vi "WASH simulated console.vi"(8 "error in (no error)":errorcluster) -> (0 "error out":errorcluster)   [LabVIEW 2015]
doc: "simulated console mimics ilustration from specification.\n\n[Covers: UI1]"
uses:
  type defs/WASH UI to CTRL commands.ctl
  type defs/WASH UI to CTRL message.ctl
  type defs/WASH CTRL to UI commands.ctl
  type defs/Wash CTRL to UI message.ctl
  type defs/WASH indicators.ctl
  type defs/WASH error levels.ctl
  type defs/WASH step selection buttons.ctl
panel:
  out "Abort":bool
  in  "Vehicle position simulation":i32(slide) scale=0.0..4.0
  out "time remaining":dbl format="%0#6.2f"
  out "vehicle out of position":bool
  out "wash indicators":T1
  out "Wash entry":bool
  in  "Start":bool
  in  "Wash step selection":T2
  # "[Covers: UI2]"
  # "[Covers: UI3]"
  # "[Covers: UI3A]\n[Covers: UI3A1]\n[Covers: UI3A2]\n[Covers: UI3A3]"
  # "[Covers: UI3B]\n[Covers: UI3B1]"
  # "[Covers: UI2A]"
  # "[Covers: UI2B]"
  # "[Covers: UI3C]\n[Covers: UI3C1]\n[Covers: UI3C2]"
  # "[Covers: UI3D]\n[Covers: UI3D1]"
  # "[Covers: UI4]"
  # "Entry"
  # "Station 1"
  # "Station 2"
  # "Station 3"
  # "Exit"
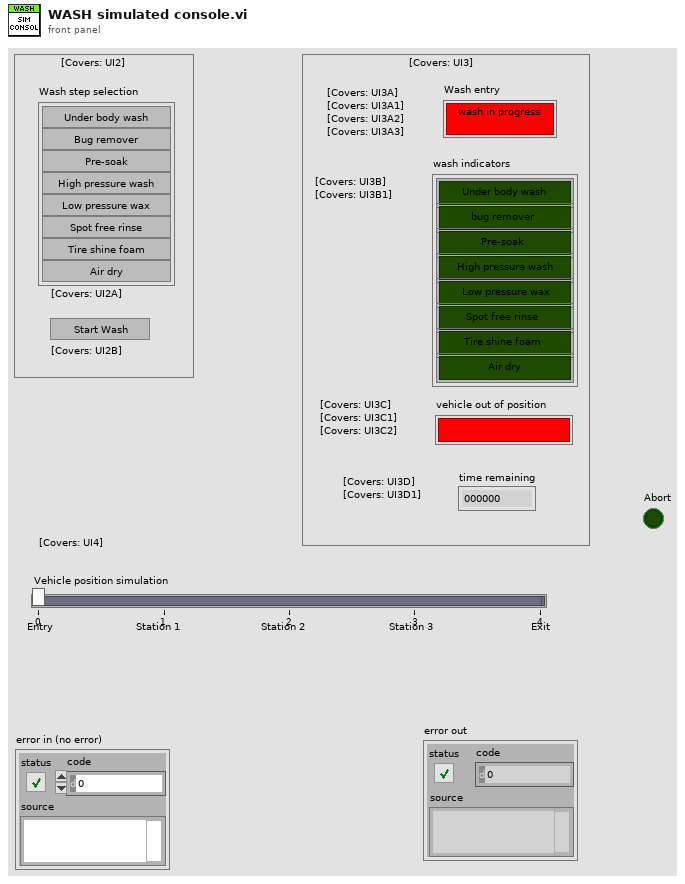
[diagram p1: front panel]
types:
  T1 = typedef "WASH indicators.ctl" = cluster{"Under body wash":bool, "bug remover":bool, "Pre-soak":bool, "High pressure wash":bool, "Low pressure wax":bool, "Spot free rinse":bool, "Tire shine foam":bool, "Air dry":bool}
  T2 = typedef "WASH step selection buttons.ctl" = cluster{"Under body wash":bool, "Bug remover":bool, "Pre-soak":bool, "High pressure wash":bool, "Low pressure wax":bool, "Spot free rinse":bool, "Tire shine foam":bool, "Air dry":bool}
  T3 = typedef "WASH UI to CTRL message.ctl" = cluster{"command":T4, "data":variant}
  T4 = typedef "WASH UI to CTRL commands.ctl" = enum16{"start button pushed", "vehicle position changed"}
  T5 = typedef "Wash CTRL to UI message.ctl" = cluster{"command":T6, "data":variant}
  T6 = typedef "WASH CTRL to UI commands.ctl" = enum16{"enable controls", "set start button value", "update vehicle out of pos", "update wash indicators", "update timing", "set vehicle position entry", "abort"}
  T7 = typedef "WASH error levels.ctl" = enum16{"minor", "wash cycle", "system"}
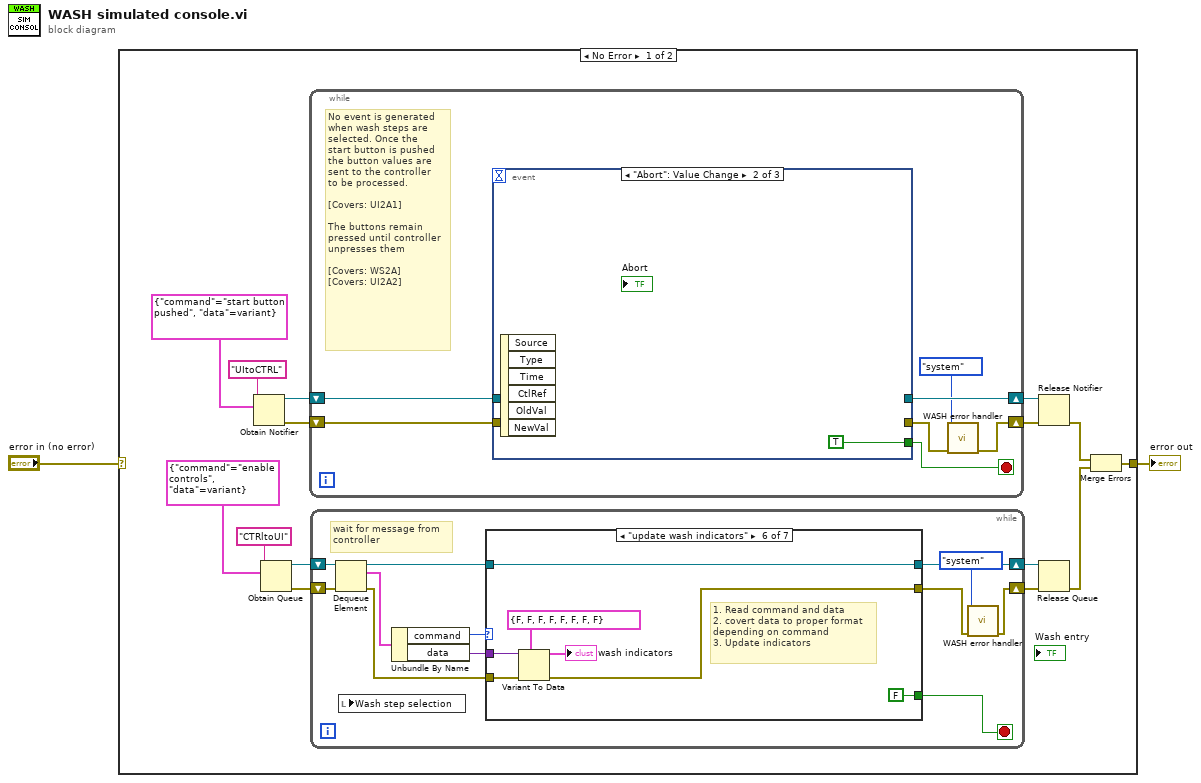
[diagram p0: block diagram]
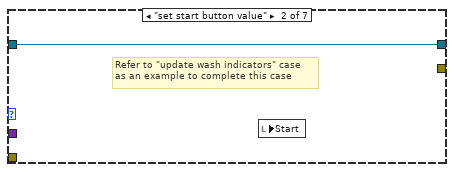
[diagram p3: hidden frame]
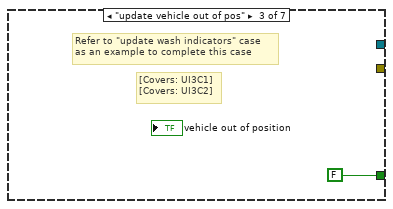
[diagram p4: hidden frame]
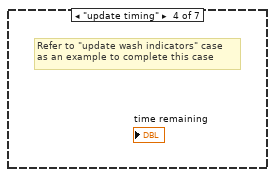
[diagram p5: hidden frame]
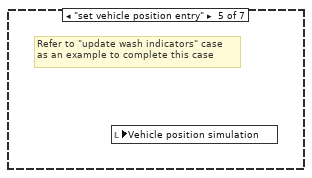
[diagram p6: hidden frame]
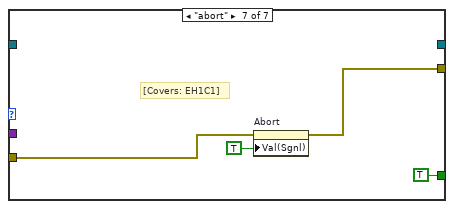
[diagram p7: hidden frame]
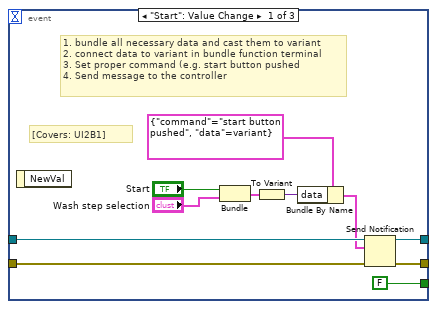
[diagram p8: hidden frame]
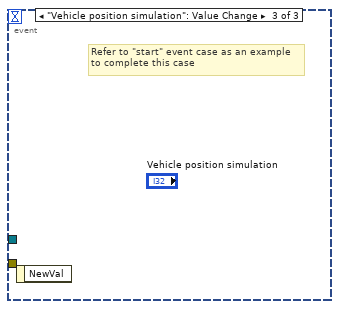
[diagram p9: hidden frame]
diagram:
  n1 = case shown="No Error" "error in (no error)" {
    selector: "error in (no error)" -> [_ w62]
    tunnel: [w3 w62] -> w1
    frame No Error {
      n2 = Obtain Notifier(name (unnamed)="UItoCTRL", notification data type=T3 {"command"=enum."start button pushed", "data"=variant} ("UI to CTRL message")) -> (notifier out=w17:refnum<notifier>, error out=w16:errorcluster)  [unwired: 2 in, 1 out]
      n3 = Obtain Queue(name (unnamed)="CTRltoUI", element data type=T5 {"command"=enum."enable controls", "data"=variant} ("CTRL to UI message")) -> (queue out=w12:refnum<queue>, error out=w11:errorcluster)  [unwired: 3 in, 1 out]
      n4 = while {
        shift-right: [w46] -> w15
        shift-left: w16 -> [w48]
        shift-right: [w47] -> w14
        shift-left: w17 -> [w49]
        stop <- w43 stop-if-true
        # "No event is generated\nwhen wash steps are\nselected. Once the\nstart button is pushed\nthe button values are\nsent to the controller\nto be processed.\n\n[Covers: UI2A1]\n\nThe buttons remain\npressed until controller\nunpresses them\n\n[Covers: WS2A]\n[Covers: UI2A2]"
        n5 = event shown="[1] \"Abort\": Value Change" {
          selector: _ -> [_ _ _]
          dyn-events: _ -> [_ _ _]
          timeout: _ -> [_ _ _]
          tunnel: w49 -> [w60 _ _]
          tunnel: [w59 _ _] -> w45
          tunnel: w48 -> [w58 _ _]
          tunnel: [w57 _ _] -> w47
          tunnel: [FALSE TRUE _] -> w43
          event "Start": Value Change {
            # "[Covers: UI2B1]"
            # "1. bundle all necessary data and cast them to variant\n2. connect data to variant in bundle function terminal\n3. Set proper command (e.g. start button pushed\n4. Send message to the controller"
            n6 = event-data() -> ()  [unwired: 1 in, 1 out]
            n7 = Bundle("Start"="Start", "Wash step selection"="Wash step selection") -> (w53:cluster{"Start":bool, "Wash step selection":T2})  [unwired: 1 in]
            n8 = To Variant(anything=w53) -> (Variant=w52:variant)
            n9 = Bundle By Name(cluster=T3 {"command"=enum."start button pushed", "data"=variant} ("notification"), "data"=w52) -> (w51:T3)
            n10 = Send Notification(notification=w51, notifier=w60, error in (no error)=w58) -> (notifier out=w57:refnum<notifier>, error out=w59:errorcluster)
          }
          event "Abort": Value Change {
            n11 = event-data() -> ()  [unwired: 1 in, 6 out]
          }
          event "Vehicle position simulation": Value Change {
            # "Refer to \"start\" event case as an example\nto complete this case"
            n12 = event-data() -> ()  [unwired: 1 in, 1 out]
          }
        }
        n13 = call "WASH error handler.vi"("error in (no error)"=w45, "error levels"=WASH_error_levels."system") -> ("error out"=w46:errorcluster)  [unwired: 7 in, 2 out]
      }
      n14 = while {
        shift-right: [w27] -> w7
        shift-left: w12 -> [w29]
        shift-right: [w20] -> w6
        shift-left: w11 -> [w28]
        stop <- w21 stop-if-true
        # "wait for message from\ncontroller"
        n15 = Dequeue Element(queue=w29, error in (no error)=w28) -> (queue out=w26:refnum<queue>, element=w25:T5, error out=w22:errorcluster)  [unwired: 1 in, 1 out]
        n16 = local read "Wash step selection"() -> ()  [unwired: 1 in]
        n17 = Unbundle By Name(w25) -> ("command"=w24:T6, "data"=w23:variant)
        n18 = case shown="\"update wash indicators\"" w24 {
          tunnel: [_ w30 _ _ _ w33 _] -> w27
          tunnel: w26 -> [_ w30 _ _ _ w33 _]
          tunnel: w23 -> [_ _ _ _ _ w38 _]
          tunnel: w22 -> [_ _ _ _ _ w37 w42]
          tunnel: [_ _ _ _ _ w34 w41] -> w19
          tunnel: [_ _ FALSE _ _ FALSE TRUE] -> w21
          frame "enable controls", Default {
            # "Refer to \"update wash indicators\" case\nas an example to complete this case"
            # "[Covers: UI2A4]"
          }
          frame "set start button value" {
            # "Refer to \"update wash indicators\" case\nas an example to complete this case"
            n19 = local read "Start"() -> ()  [unwired: 1 in]
          }
          frame "update vehicle out of pos" {
            # "Refer to \"update wash indicators\" case\nas an example to complete this case"
            # "[Covers: UI3C1]\n[Covers: UI3C2]"
          }
          frame "update timing" {
            # "Refer to \"update wash indicators\" case\nas an example to complete this case"
          }
          frame "set vehicle position entry" {
            # "Refer to \"update wash indicators\" case\nas an example to complete this case"
            n20 = local read "Vehicle position simulation"() -> ()  [unwired: 1 in]
          }
          frame "update wash indicators" {
            # "1. Read command and data\n2. covert data to proper format\ndepending on command\n3. Update indicators"
            n21 = Variant To Data(error in=w37, type=T1 {"Under body wash"=FALSE, "bug remover"=FALSE, "Pre-soak"=FALSE, "High pressure wash"=FALSE, "Low pressure wax"=FALSE, "Spot free rinse"=FALSE, "Tire shine foam"=FALSE, "Air dry"=FALSE} ("wash indicators"), Variant=w38) -> (data=→"wash indicators":T1, error out=w34:errorcluster)
          }
          frame "abort" {
            # "[Covers: EH1C1]"
            n22 = property on="Abort" class="Bool (strict)"(error in=w42, "Val(Sgnl)"=TRUE ("Value (Signaling)")) -> (error out=w41:errorcluster)  [unwired: 1 in, 1 out]
          }
        }
        n23 = call "WASH error handler.vi"("error in (no error)"=w19, "error levels"=WASH_error_levels."system") -> ("error out"=w20:errorcluster)  [unwired: 7 in, 2 out]
      }
      n24 = Release Notifier(notifier=w14, error in (no error)=w15) -> (error out=w5:errorcluster)  [unwired: 3 out]
      n25 = Release Queue(queue=w7, error in (no error)=w6) -> (error out=w4:errorcluster)  [unwired: 1 in, 2 out]
      n26 = Merge Errors(w5, w4) -> (w3:errorcluster)
    }
    frame Error {
    }
  }
  "error out" <- w1
